vi "GSP_hexstringtonum.vi"(3 "low 16 (hex)":string, 5 "high 16 (hex)":string) -> (0 "Low Word":u16, 1 "#":i32, 2 "High Word":u16)   [LabVIEW 2015]
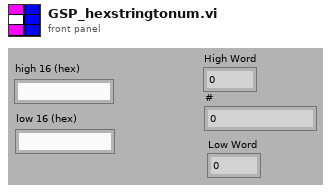
[diagram p1: front panel]
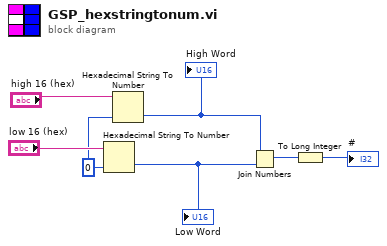
[diagram p0: block diagram]
diagram:
  w1 = u16 0 ("default (0 U32)")
  n1 = Hexadecimal String To Number(string="low 16 (hex)", default (0uL)=w1) -> (number=w2:u16)  [unwired: 1 in, 1 out]
  "Low Word" <- w2
  n2 = Hexadecimal String To Number(string="high 16 (hex)", default (0uL)=w1) -> (number=w3:u16)  [unwired: 1 in, 1 out]
  "High Word" <- w3
  n3 = Join Numbers(hi=w3, lo=w2) -> ((hi.lo)=w4:u32)
  n4 = To Long Integer(number=w4) -> (32bit integer=→"#":i32)
